vi "run.vi"(8 "error in (no error)":errorcluster, 11 "Monochromator in":refnum<class "Monochromator.lvclass">) -> (0 "error out":errorcluster, 3 "Monochromator out":refnum<class "Monochromator.lvclass">)   [LabVIEW 2016, in "Monochromator.lvclass"]
uses:
  Monochromator.lvclass
  Typedefs/wavelength.ctl
  Typedefs/GratingType.ctl
  Typedefs/DeviceStatus.ctl
  Monochromator.lvclass/Monochromator.ctl
  Typedefs/slit.ctl
  Typedefs/SlitType.ctl
  Typedefs/slitWidth.ctl
  MonoCommunicator/MonoCommunicator.lvclass
panel:
  out "DeviceStatus":T1
  out "Exit Slit":dbl
  out "Entrance slit":dbl
  out "Status":string
  out "Emulating":bool
  out "Initialized":bool
  out "wavelength":T2
  out "GratingType":T3=enum."Red"
  # "Status"
  # "Grating"
  # "Wavelength"
  # "Slit Width"
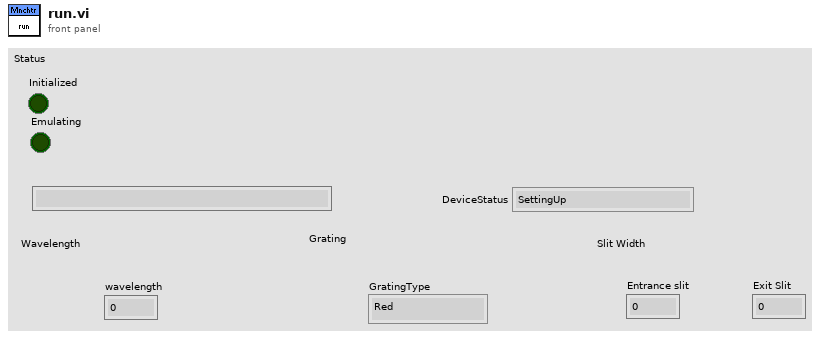
[diagram p1: front panel]
types:
  T1 = typedef "DeviceStatus.ctl" = enum16{"SettingUp", "Ready", "Offline", "Fault"}
  T2 = typedef "wavelength.ctl" = dbl
  T3 = typedef "GratingType.ctl" = enum16{"NoGrating", "Red", "Blue", "Mirror"}
  T4 = typedef "slit.ctl" = cluster{"SlitType":T5, "Width":T6}
  T5 = typedef "SlitType.ctl" = enum16{"Front Entrance", "Side Entrance", "Front Exit", "Side Exit", "First Intermediate", "Second Intermediate"}
  T6 = typedef "slitWidth.ctl" = dbl
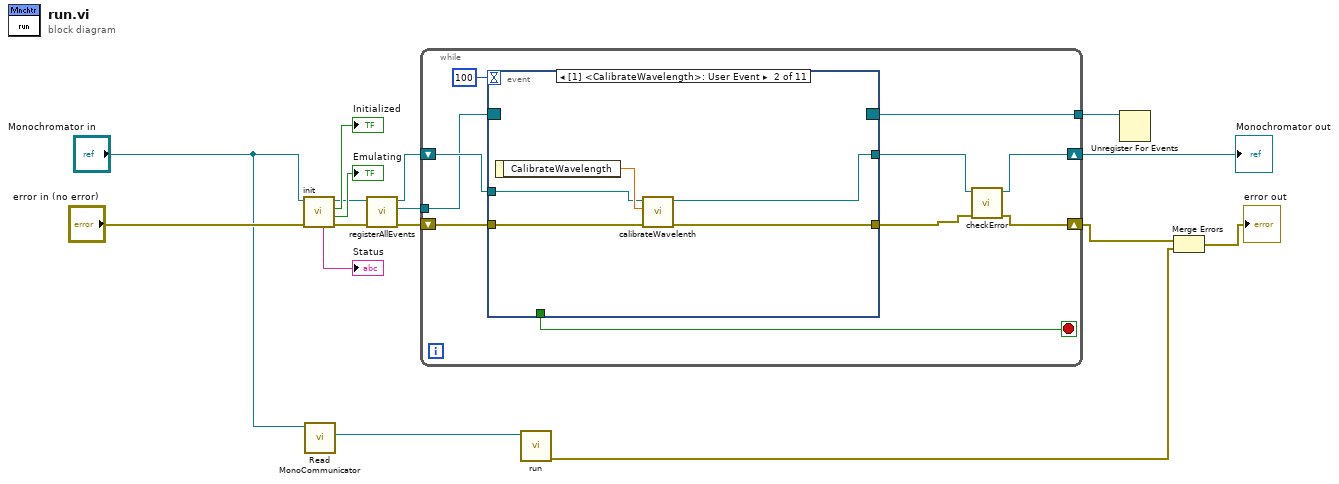
[diagram p0: block diagram]
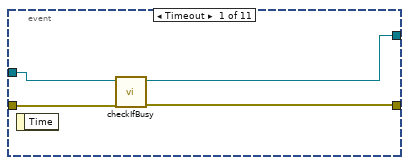
[diagram p2: hidden frame]
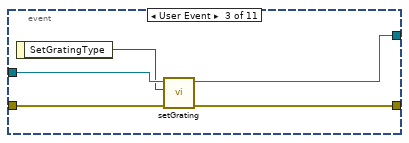
[diagram p3: hidden frame]
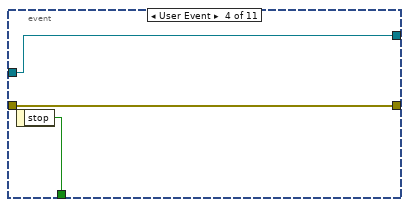
[diagram p4: hidden frame]
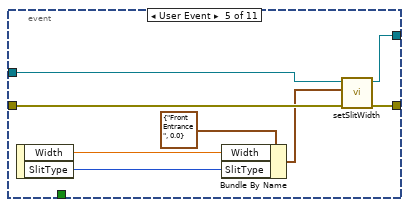
[diagram p5: hidden frame]
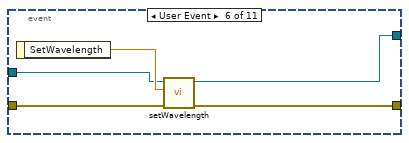
[diagram p6: hidden frame]
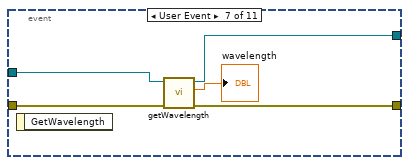
[diagram p7: hidden frame]
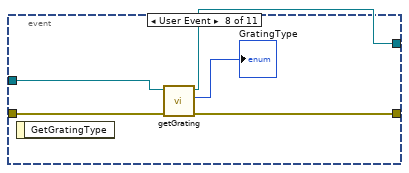
[diagram p8: hidden frame]
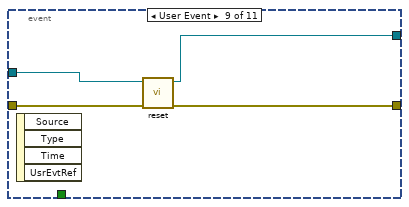
[diagram p9: hidden frame]
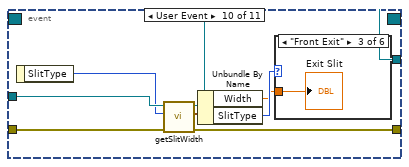
[diagram p10: hidden frame]
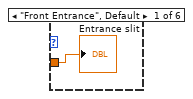
[diagram p11: hidden frame]
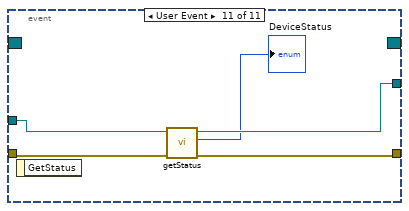
[diagram p16: hidden frame]
diagram:
  n1 = call "init.vi"("error in (no error)"="error in (no error)", "Monochromator in"="Monochromator in") -> ("error out"=w9:errorcluster, "Emulating"=→"Emulating":bool, "Initialized"=→"Initialized":bool, "Monochromator out"=w11:refnum<class "Monochromator.lvclass">, "Status"=→"Status":string)  [unwired: 5 in]
  n2 = call "Read MonoCommunicator.vi"("Monochromator in"="Monochromator in") -> ("MonoCommunicator.lvclass"=w5:refnum<class "MonoCommunicator.lvclass">)  [unwired: 8 in, 2 out]
  n3 = call "registerAllEvents.vi"("error in (no error)"=w9, "Monochromator in"=w11) -> ("error out"=w8:errorcluster, "AllEventsRegRefnum"=w7:refnum<event-registration>, "Monochromator out"=w10:refnum<class "Monochromator.lvclass">)  [unwired: 7 in]
  n4 = while {
    tunnel: w7 -> [w24]
    tunnel: [w21] -> w1
    shift-right: [w17] -> w12
    shift-left: w10 -> [w25]
    shift-right: [w19] -> w3
    shift-left: w8 -> [w23]
    stop <- w22 stop-if-true
    n5 = event shown="[1] <CalibrateWavelength>: User Event" {
      selector: w24 -> [_ _ _ _ _ _ _ _ _ _ _]
      dyn-events: [_ _ _ _ _ _ _ _ _ _ _] -> w21
      timeout: 100 -> [_ _ _ _ _ _ _ _ _ _ _]
      tunnel: w25 -> [w30 w32 w38 w42 w51 w55 w61 w64 w70 w78 w84]
      tunnel: [w27 w33 w37 w42 w50 w54 w58 w62 w67 w74 w83] -> w18
      tunnel: w23 -> [w29 w34 w40 w41 w49 w53 w60 w66 w69 w76 w85]
      tunnel: [w28 w31 w39 w41 w48 w52 w59 w65 w68 w75 w82] -> w20
      tunnel: [_ _ _ w43 _ _ _ _ _ _ _] -> w22
      event Timeout {
        n6 = event-data() -> ()  [unwired: 1 in, 1 out]
        n7 = call "checkIfBusy.vi"("error in (no error)"=w29, "Monochromator in"=w30) -> ("error out"=w28:errorcluster, "Monochromator out"=w27:refnum<class "Monochromator.lvclass">)  [unwired: 8 in]
      }
      event User Event {
        n8 = event-data() -> ("CalibrateWavelength"=w35:T2)  [unwired: 1 in]
        n9 = call "calibrateWavelenth.vi"("error in (no error)"=w34, "wavelength"=w35, "Monochromator in"=w32) -> ("error out"=w31:errorcluster, "Monochromator out"=w33:refnum<class "Monochromator.lvclass">)  [unwired: 7 in]
      }
      event User Event {
        n10 = event-data() -> ("SetGratingType"=w36:T3)  [unwired: 1 in]
        n11 = call "setGrating.vi"("error in (no error)"=w40, "GratingType"=w36, "Monochromator in"=w38) -> ("error out"=w39:errorcluster, "Monochromator out"=w37:refnum<class "Monochromator.lvclass">)  [unwired: 7 in]
      }
      event User Event {
        n12 = event-data() -> ("stop"=w43:bool)  [unwired: 1 in]
      }
      event User Event {
        n13 = event-data() -> ("Width"=w46:T6, "SlitType"=w45:T5)  [unwired: 1 in]
        n14 = Bundle By Name(cluster=T4 {"SlitType"=enum."Front Entrance", "Width"=0.0} ("position"), "Width"=w46, "SlitType"=w45) -> (w44:T4)
        n15 = call "setSlitWidth.vi"("error in (no error)"=w49, "position"=w44, "Monochromator in"=w51) -> ("error out"=w48:errorcluster, "Monochromator out"=w50:refnum<class "Monochromator.lvclass">)  [unwired: 7 in]
      }
      event User Event {
        n16 = event-data() -> ("SetWavelength"=w56:T2)  [unwired: 1 in]
        n17 = call "setWavelength.vi"("error in (no error)"=w53, "wavelength"=w56, "Monochromator in"=w55) -> ("error out"=w52:errorcluster, "Monochromator out"=w54:refnum<class "Monochromator.lvclass">)  [unwired: 7 in]
      }
      event User Event {
        n18 = event-data() -> ()  [unwired: 1 in, 1 out]
        n19 = call "getWavelength.vi"("error in (no error)"=w60, "Monochromator in"=w61) -> ("error out"=w59:errorcluster, "wavelength"=→"wavelength":T2, "Monochromator out"=w58:refnum<class "Monochromator.lvclass">)  [unwired: 7 in]
      }
      event User Event {
        n20 = event-data() -> ()  [unwired: 1 in, 1 out]
        n21 = call "getGrating.vi"("error in (no error)"=w66, "Monochromator in"=w64) -> ("error out"=w65:errorcluster, "GratingType"=→"GratingType":T3, "Monochromator out"=w62:refnum<class "Monochromator.lvclass">)  [unwired: 7 in]
      }
      event User Event {
        n22 = event-data() -> ()  [unwired: 1 in, 4 out]
        n23 = call "reset.vi"("error in (no error)"=w69, "Monochromator in"=w70) -> ("error out"=w68:errorcluster, "Monochromator out"=w67:refnum<class "Monochromator.lvclass">)  [unwired: 8 in]
      }
      event User Event {
        n24 = event-data() -> ("SlitType"=w77:T5)  [unwired: 1 in]
        n25 = call "getSlitWidth.vi"("error in (no error)"=w76, "SlitType in"=w77, "Monochromator in"=w78) -> ("error out"=w75:errorcluster, "position"=w73:T4, "Monochromator out"=w74:refnum<class "Monochromator.lvclass">)  [unwired: 6 in]
        n26 = Unbundle By Name(w73) -> ("Width"=w71:T6, "SlitType"=w72:T5)
        n27 = case shown="\"Front Exit\"" w72 {
          tunnel: w71 -> [w79 _ w80 _ _ _]
          frame "Front Entrance", Default {
            "Entrance slit" <- w79
          }
          frame "Side Entrance" {
          }
          frame "Front Exit" {
            "Exit Slit" <- w80
          }
          frame "Side Exit" {
          }
          frame "First Intermediate" {
          }
          frame "Second Intermediate" {
          }
        }
      }
      event User Event {
        n28 = event-data() -> ()  [unwired: 1 in, 1 out]
        n29 = call "getStatus.vi"("error in (no error)"=w85, "Monochromator in"=w84) -> ("error out"=w82:errorcluster, "DeviceStatus"=→"DeviceStatus":T1, "Monochromator out"=w83:refnum<class "Monochromator.lvclass">)  [unwired: 7 in]
      }
    }
    n30 = call "checkError.vi"("error in (no error)"=w20, "Monochromator in"=w18) -> ("error out"=w19:errorcluster, "Monochromator out"=w17:refnum<class "Monochromator.lvclass">)  [unwired: 8 in]
  }
  "Monochromator out" <- w12
  n31 = call "run.vi"("MonoCommunicator in"=w5) -> ("error out"=w2:errorcluster)  [unwired: 9 in, 1 out]
  n32 = Unregister For Events(event registration refnum=w1) -> ()  [unwired: 1 in, 1 out]
  n33 = Merge Errors(w3, w2) -> (→"error out":errorcluster)
